vi "Test Configuration - NF.vi"(8 "error in (no error)":errorcluster, 10 "Test Configuration":T1 {"Frequency List (Hz)" format="%.3p"; "NF DUT Type" items=["Amplifier", "Downconverter", "Upconverter"]; "Y-Factor Mode" items=["Measure", "Calibrate"]; "Noise Source"."Noise Source Type" items=["External Noise Source", "RF Signal Generator"]; "Noise Source"."ENR (dB)" format="%.2g"; "Noise Source"."ENR Freq (Hz)" format="%.3p"; "Noise Source"."Off Temperature (K)" format="%.2f"; "Noise Source"."Cold Temperature (K)" format="%.2f"; "Averaging"."Enabled" items=["False", "True"]; "Measurement Interval (s)" format="%.2p"; "Measurement Bandwidth (Hz)" format="%.3p"}, 11 "RFmx Session in":refnum<k21>) -> (0 "error out":errorcluster, 3 "RFmx Session out":refnum<k21>)   [LabVIEW 2023]
uses:
  Controls/Test Config - NF.ctl
  <resource>/objmgr/RFmxSpecAn.rc
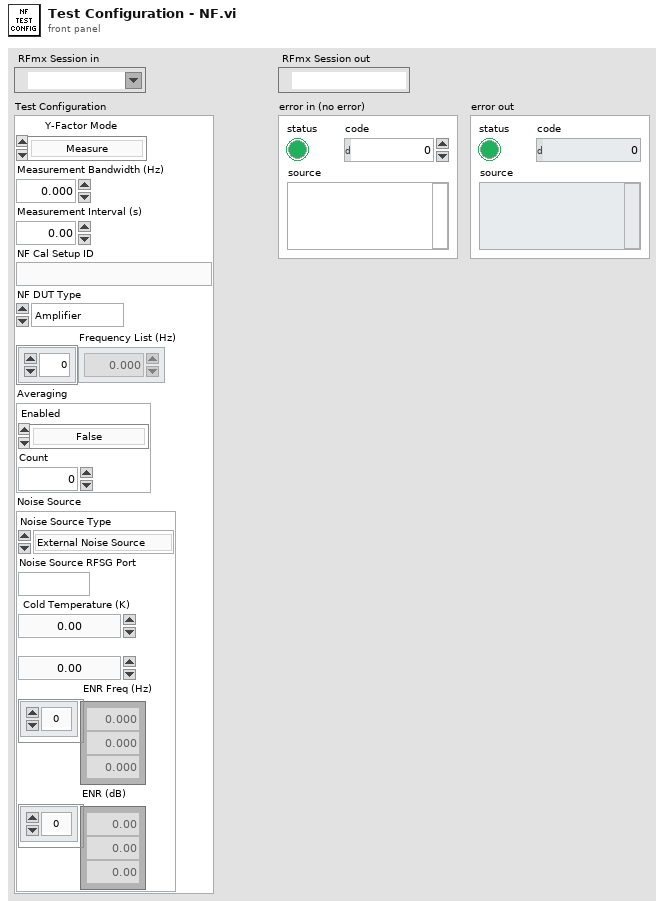
[diagram p1: front panel]
types:
  T1 = typedef "Test Config - NF.ctl" = cluster{"Y-Factor Mode":i32, "Measurement Bandwidth (Hz)":dbl, "Measurement Interval (s)":dbl, "NF Cal Setup ID":string, "NF DUT Type":i32, "Frequency List (Hz)":dbl[], "Averaging":cluster{"Enabled":i32, "Count":i32}, "Noise Source":cluster{"Noise Source Type":i32, "Noise Source RFSG Port":string, "Cold Temperature (K)":dbl, "Off Temperature (K)":dbl, "ENR Freq (Hz)":dbl[], "ENR (dB)":dbl[]}}
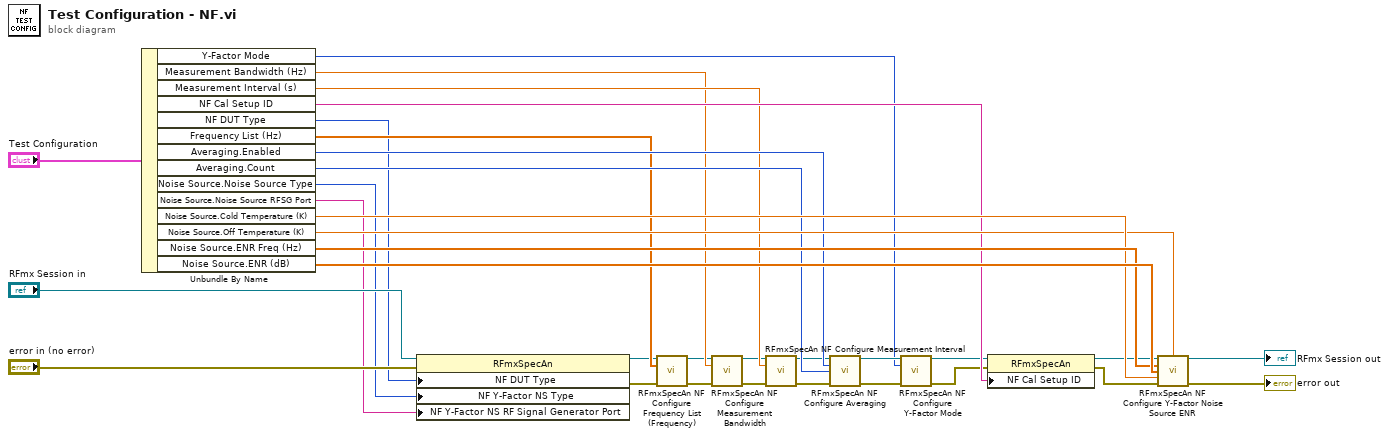
[diagram p0: block diagram]
diagram:
  n1 = Unbundle By Name("Test Configuration") -> ("Y-Factor Mode"=w24:i32, "Measurement Bandwidth (Hz)"=w20:dbl, "Measurement Interval (s)"=w21:dbl, "NF Cal Setup ID"=w25:string, "NF DUT Type"=w17:i32, "Frequency List (Hz)"=w19:dbl[], "Averaging.Enabled"=w23:i32, "Averaging.Count"=w22:i32, "Noise Source.Noise Source Type"=w18:i32, "Noise Source.Noise Source RFSG Port"=w1:string, "Noise Source.Cold Temperature (K)"=w27:dbl, "Noise Source.Off Temperature (K)"=w26:dbl, "Noise Source.ENR Freq (Hz)"=w28:dbl[], "Noise Source.ENR (dB)"=w29:dbl[])
  n2 = property class="RFmxSpecAn"(reference="RFmx Session in", error in="error in (no error)", "NF DUT Type"=w17, "NF Y-Factor NS Type"=w18, "NF Y-Factor NS RF Signal Generator Port"=w1) -> (reference out=w10:refnum<k21>, error out=w11:errorcluster)
  n3 = call <vilib>:"RFmxSpecAn NF Configure Frequency List (Frequency).vi"("Instrument Handle In"=w10, "Frequency List (Hz)"=w19, "error in (no error)"=w11) -> ("Instrument Handle Out"=w4:refnum<k21>, "error out"=w7:errorcluster)  [unwired: 11 in]
  n4 = call <vilib>:"RFmxSpecAn NF Configure Measurement Bandwidth.vi"("Instrument Handle In"=w4, "Measurement Bandwidth (Hz)"=w20, "error in (no error)"=w7) -> ("Instrument Handle Out"=w5:refnum<k21>, "error out"=w6:errorcluster)  [unwired: 11 in]
  n5 = call <vilib>:"RFmxSpecAn NF Configure Measurement Interval.vi"("Instrument Handle In"=w5, "Measurement Interval (s)"=w21, "error in (no error)"=w6) -> ("Instrument Handle Out"=w8:refnum<k21>, "error out"=w9:errorcluster)  [unwired: 11 in]
  n6 = call <vilib>:"RFmxSpecAn NF Configure Averaging.vi"("Instrument Handle In"=w8, "Averaging Enabled"=w23, "Averaging Count"=w22, "error in (no error)"=w9) -> ("Instrument Handle Out"=w30:refnum<k21>, "error out"=w31:errorcluster)  [unwired: 10 in]
  n7 = call <vilib>:"RFmxSpecAn NF Configure Y-Factor Mode.vi"("Instrument Handle In"=w30, "Y-Factor Mode"=w24, "error in (no error)"=w31) -> ("Instrument Handle Out"=w14:refnum<k21>, "error out"=w12:errorcluster)  [unwired: 11 in]
  n8 = property class="RFmxSpecAn"(reference=w14, error in=w12, "NF Cal Setup ID"=w25) -> (reference out=w15:refnum<k21>, error out=w13:errorcluster)
  n9 = call <vilib>:"RFmxSpecAn NF Configure Y-Factor Noise Source ENR.vi"("Instrument Handle In"=w15, "Off Temperature (K)"=w26, "ENR Freq (Hz)"=w28, "ENR (dB)"=w29, "Cold Temperature (K)"=w27, "error in (no error)"=w13) -> ("Instrument Handle Out"=→"RFmx Session out":refnum<k21>, "error out"=→"error out":errorcluster)  [unwired: 8 in]
